vi "Broadcast Boolean.vi"(8 "error in (no error)":errorcluster, 10 "Boolean":bool, 11 "Alternative Example Sink in":refnum<class "Alternative Example Sink.lvclass">) -> (0 "error out":errorcluster, 3 "Alternative Example Sink out":refnum<class "Alternative Example Sink.lvclass">)   [LabVIEW 2016, in "Alternative Example Sink.lvlib" / "Alternative Example Sink.lvclass"]
uses:
  Alternative Example Sink.lvclass
  C:/Projects/Shared Libraries/Event Actors/Event Sink/Event Sink.lvclass
  Example Source/Example Events/Boolean Event.lvclass
  C:/Projects/Shared Libraries/Event Actors/Event/Event.lvclass
  Example Source/Example Events/Boolean Event.lvclass/Boolean Event.ctl
  Event Sink/Event Sink.lvclass
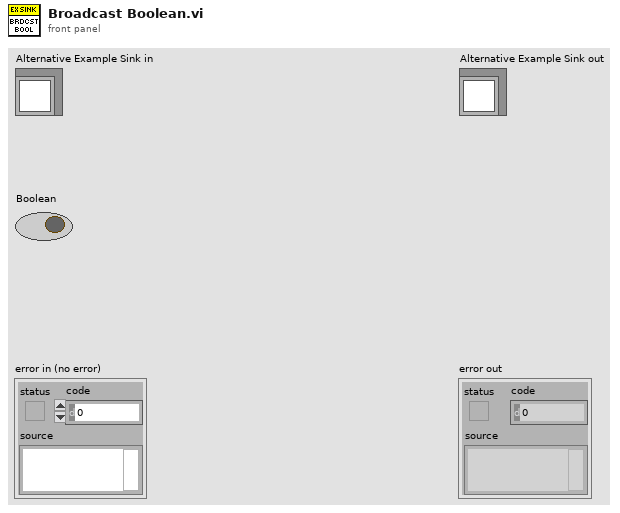
[diagram p1: front panel]
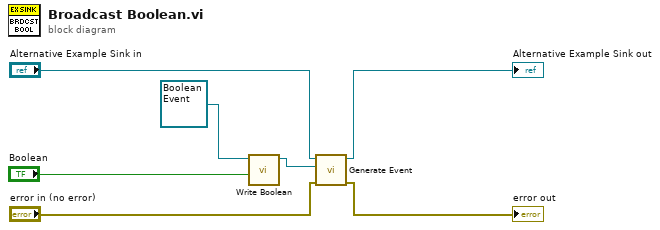
[diagram p0: block diagram]
diagram:
  n1 = call "Write Boolean.vi"("Boolean"="Boolean", "Boolean Event in"=refnum<class "Boolean Event.lvclass"> refnum ("Example Source.lvlib:Boolean Event.lvclass")) -> ("Boolean Event out"=w1:refnum<class "Boolean Event.lvclass">)  [unwired: 9 in]
  n2 = call "Generate Event.vi"("error in (no error)"="error in (no error)", "Event Data"=w1, "Event Sink in"="Alternative Example Sink in") -> ("error out"=→"error out":errorcluster, "Event Sink out"=→"Alternative Example Sink out":refnum<class "Alternative Example Sink.lvclass">)  [unwired: 7 in]
